vi "Get Owning Ballard ARINC-429 Custom Device.vi"(8 "error in":errorcluster, 11 "item ref in":T1 format="%.0x") -> (0 "error out":errorcluster, 2 "owning Ballard ARINC-429 custom device":T1=18446744073709551615 format="%.0x", 3 "item ref out":T1 format="%.0x")   [LabVIEW 2020, in "Communication Bus Template Scripting.lvlib"]
uses:
  Communication Bus Template Scripting.lvlib
  Constants.vi
  <vilib>/NI VeriStand/Custom Device Tools/Custom Device Utility Library/Custom Device Utility Library.lvlib
  <vilib>/NI VeriStand/Custom Device Tools/Custom Device Utility Library/Search Direction.ctl
  <vilib>/NI VeriStand/Custom Device Tools/Custom Device Utility Library/NI VeriStand - Search for Item by GUID.vi
  <vilib>/NI VeriStand/Custom Device API/Custom Device Item Ref.ctl
  <vilib>/NI VeriStand/Custom Device API/Custom Device API.lvlib
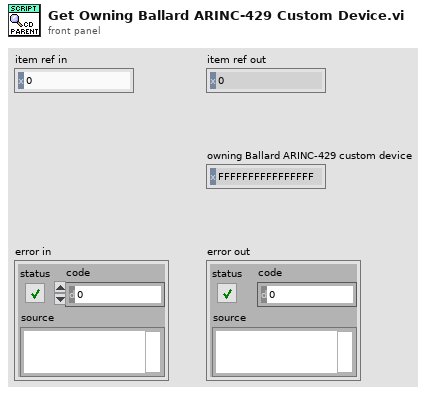
[diagram p1: front panel]
types:
  T1 = typedef "Custom Device API.lvlib/Custom Device Item Ref.ctl" = u64
  T2 = typedef "Custom Device Utility Library.lvlib/Search Direction.ctl" = enum16{"Down", "Up"}
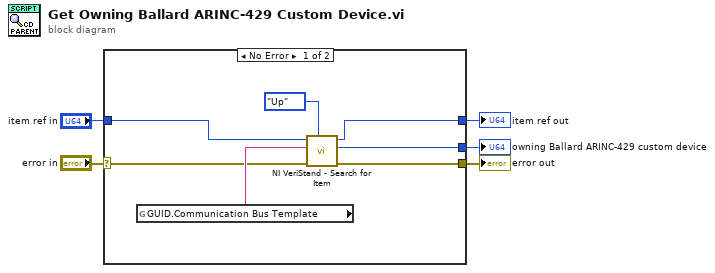
[diagram p0: block diagram]
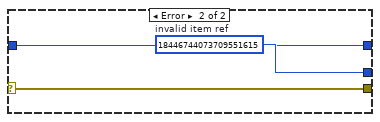
[diagram p2: hidden frame]
diagram:
  n1 = case shown="No Error" "error in" {
    selector: "error in" -> [w9 w15]
    tunnel: "item ref in" -> [w10 w13]
    tunnel: [w8 w14] -> w4
    tunnel: [w7 w15] -> w2
    tunnel: [w6 w13] -> w1
    frame No Error {
      n2 = global read "Constants.vi" "GUID.Communication Bus Template"() -> (w12:string)
      n3 = call-poly <vilib>:"NI VeriStand - Search for Item.vi"("Direction (Down)"=Search_Direction."Up", "error in"=w9, "Item GUID"=w12, "Section Ref in"=w10) -> ("error out"=w7:errorcluster, "Item Ref"=w8:T1, "Section Ref out"=w6:T1)  [unwired: 4 in, 1 out]
    }
    frame Error {
      w14 = T1 18446744073709551615  # invalid item ref
    }
  }
  "owning Ballard ARINC-429 custom device" <- w4
  "error out" <- w2
  "item ref out" <- w1
